vi "Write Serialisation.vi"(8 "error in (no error)":errorcluster, 10 "Serialisation":T1, 11 "CommHandlerBase in":refnum<class "CommHandlerBase.lvclass">) -> (0 "error out":errorcluster, 3 "CommHandlerBase out":refnum<class "CommHandlerBase.lvclass">)   [LabVIEW 2020, in "wamplv.lvlib" / "CommHandlerBase.lvclass"]
uses:
  CommHandlerBase.lvclass
  WAMP Client/API/TypeDefs/Serialisation.ctl
  CommHandlerBase.lvclass/CommHandlerBase.ctl
  WAMP Client/WAMP Client.lvclass
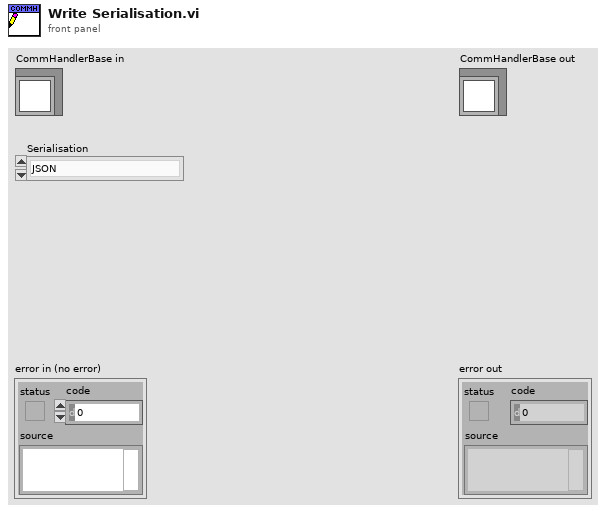
[diagram p1: front panel]
types:
  T1 = typedef "wamplv.lvlib/WAMP Client.lvclass/Serialisation.ctl" = enum16{"JSON", "MessagePack"}
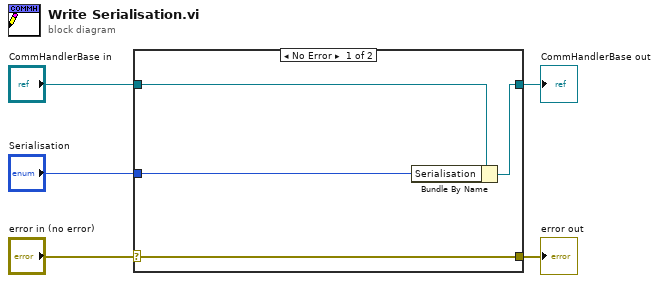
[diagram p0: block diagram]
diagram:
  n1 = case shown="No Error" "error in (no error)" {
    selector: "error in (no error)" -> [w9 w10]
    tunnel: [w9 w10] -> w4
    tunnel: [w7 w11] -> w2
    tunnel: "CommHandlerBase in" -> [w8 w11]
    tunnel: "Serialisation" -> [w6 _]
    frame No Error {
      n2 = Bundle By Name(cluster=w8, "Serialisation"=w6) -> (w7:refnum<class "CommHandlerBase.lvclass">)
    }
    frame Error {
    }
  }
  "error out" <- w4
  "CommHandlerBase out" <- w2
